vi "Convert to RelativePath.vi"(8 "error in (no error)":errorcluster caption="错误输入（无错误）", 11 "VI Path":path) -> (0 "error out":errorcluster caption="错误输出", 3 "RelativePath":string)   [LabVIEW 2016, in "PanelRootNode.lvclass"]
uses:
  PanelRootNode.lvclass
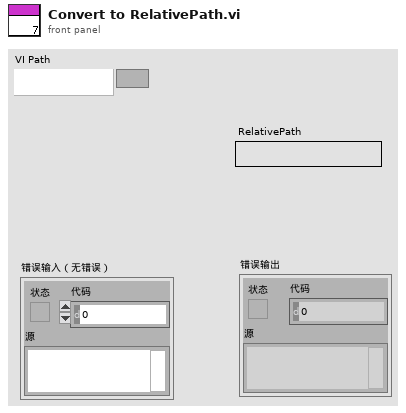
[diagram p1: front panel]
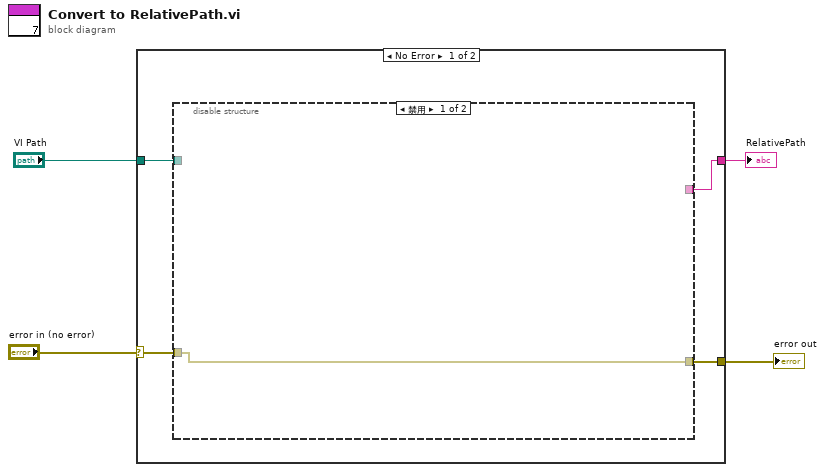
[diagram p0: block diagram]
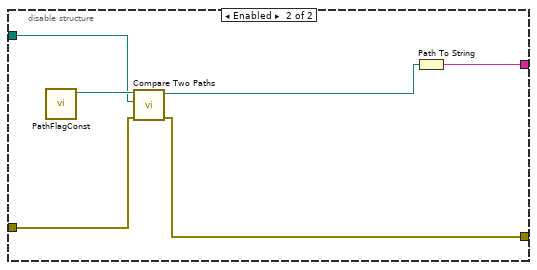
[diagram p2: hidden frame]
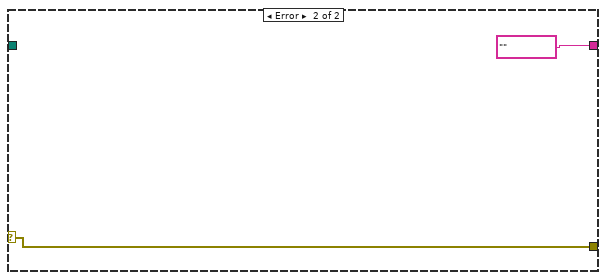
[diagram p3: hidden frame]
diagram:
  n1 = case shown="No Error" "error in (no error)" {
    selector: "error in (no error)" -> [w7 w17]
    tunnel: [w8 w17] -> w4
    tunnel: "VI Path" -> [w6 _]
    tunnel: [w5 ""] -> w1
    frame No Error {
      n2 = disable-structure shown="禁用" {
        disable-tunnel: [w9 w10] -> w8
        disable-tunnel: w7 -> [w9 w11]
        disable-tunnel: w6 -> [_ w14]
        disable-tunnel: [_ w12] -> w5
        frame Disabled {
        }
        frame Enabled {
          n3 = call "PathFlagConst.vi"() -> ("路径"=w15:path)  [unwired: 11 in]
          n4 = call <vilib>:"Compare Two Paths.vi"("error in (no error)"=w11, "Path 2"=w14, "Path 1"=w15) -> ("error out"=w10:errorcluster, "Relative Path from 1 to 2"=w13:path)  [unwired: 5 in, 2 out]
          n5 = Path To String(path=w13) -> (string=w12:string)
        }
      }
    }
    frame Error {
    }
  }
  "error out" <- w4
  "RelativePath" <- w1
